vi "Create Trace.vi"(4 "Trace Payload":string, 6 "Trace Payload Type":string, 7 "Trace Source":string, 8 "Trace Level":T1(ring)=enum."Debug", 9 "Trace Message":string, 10 "Instance Name":string, 11 "System Name":string) -> (3 "Trace":refnum<class "Trace.lvclass">)   [LabVIEW 2014, in "Robot Actor Framework.lvlib" / "Trace.lvlib" / "Trace.lvclass"]
uses:
  Trace Class/Trace.lvclass
panel:
  out "error out":errorcluster
  in  "error in (no error)":errorcluster
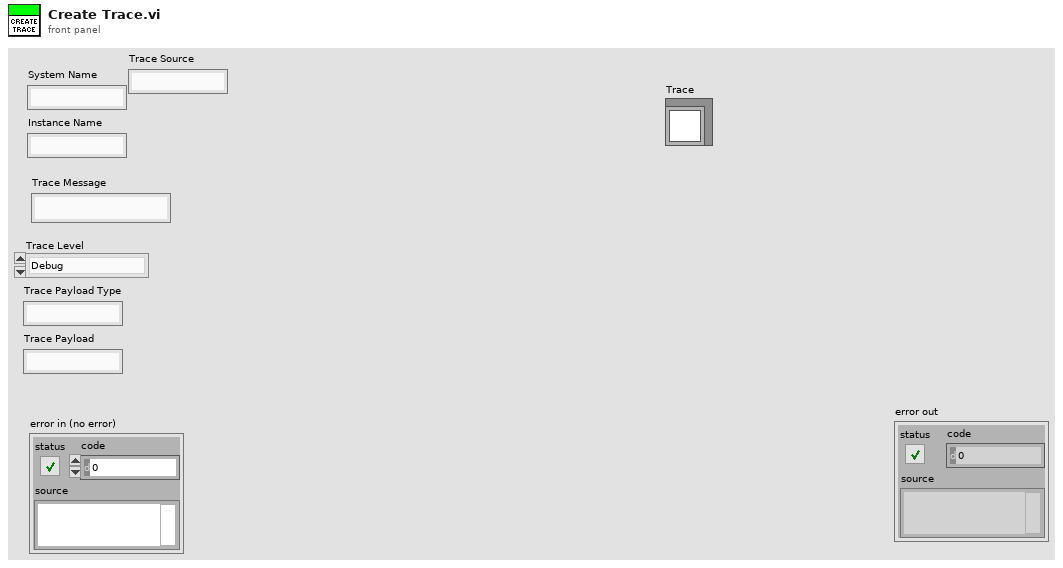
[diagram p1: front panel]
types:
  T1 = enum16{"Critical", "Error", "Warning", "Informational", "Debug"}
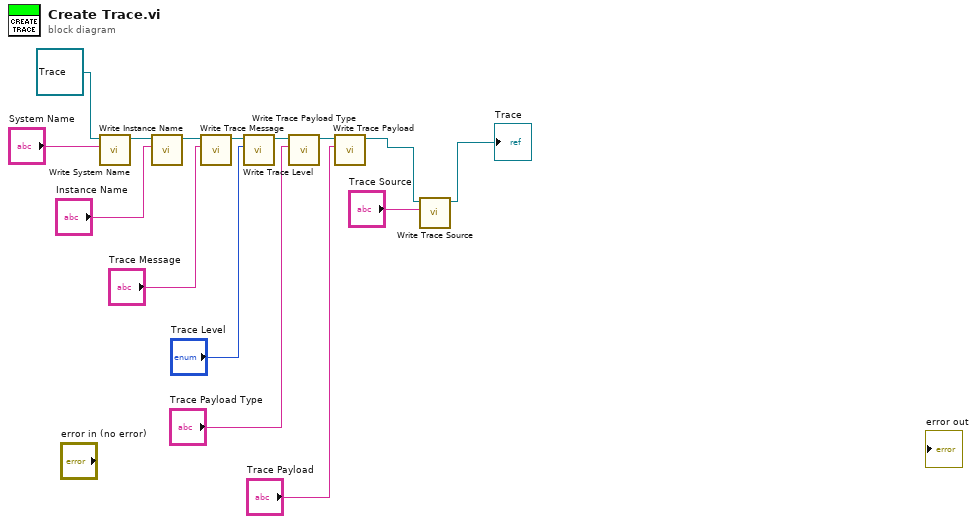
[diagram p0: block diagram]
diagram:
  n1 = call-dynamic "Write System Name.vi"("System Name (Inst)"="System Name", "Trace in"=refnum<class "Trace.lvclass"> refnum ("Robot Actor Framework.lvlib:Trace.lvlib:Trace.lvclass")) -> ("Trace out"=w14:refnum<class "Trace.lvclass">)  [unwired: 8 in, 1 out]
  n2 = call-dynamic "Write Instance Name.vi"("Instance Name"="Instance Name", "Trace in"=w14) -> ("Trace out"=w9:refnum<class "Trace.lvclass">)  [unwired: 8 in, 1 out]
  n3 = call-dynamic "Write Trace Message.vi"("Trace Message"="Trace Message", "Trace in"=w9) -> ("Trace out"=w8:refnum<class "Trace.lvclass">)  [unwired: 8 in, 1 out]
  n4 = call-dynamic "Write Trace Level.vi"("Trace Level"="Trace Level", "Trace in"=w8) -> ("Trace out"=w13:refnum<class "Trace.lvclass">)  [unwired: 8 in, 1 out]
  n5 = call-dynamic "Write Trace Payload Type.vi"("Trace Payload Type"="Trace Payload Type", "Trace in"=w13) -> ("Trace out"=w12:refnum<class "Trace.lvclass">)  [unwired: 8 in, 1 out]
  n6 = call-dynamic "Write Trace Payload.vi"("Trace Payload"="Trace Payload", "Trace in"=w12) -> ("Trace out"=w3:refnum<class "Trace.lvclass">)  [unwired: 8 in, 1 out]
  n7 = call-dynamic "Write Trace Source.vi"("Trace Source"="Trace Source", "Trace in"=w3) -> ("Trace out"=→"Trace":refnum<class "Trace.lvclass">)  [unwired: 8 in, 1 out]
